vi "Practica_01.vi"() -> ()   [LabVIEW 2020]
panel:
  in  "stop":bool
  out "Grafica Filtro EMA":dbl(graph)
  out "Voltaje vs Tiempo":dbl[](graph)
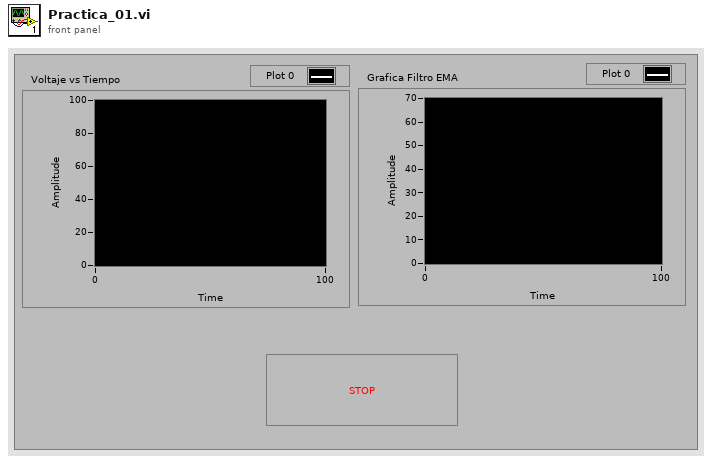
[diagram p1: front panel]
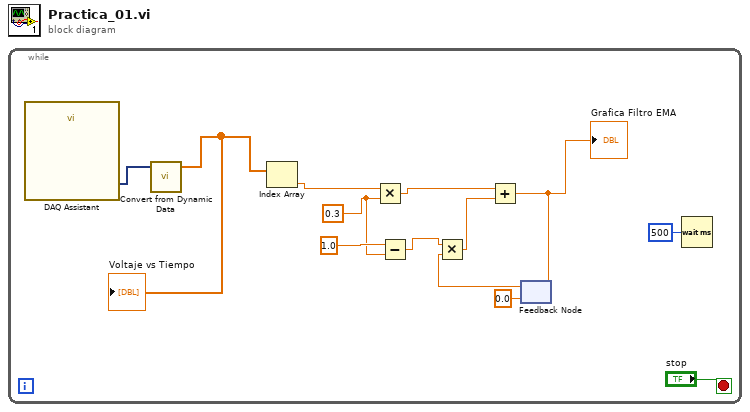
[diagram p0: block diagram]
diagram:
  n1 = while {
    stop <- "stop" stop-if-true
    w7 = 0.3 ("y")
    n2 = call "DAQ Assistant"() -> ("data"=w2:dynamicdata)  [unwired: 17 in, 2 out]
    n3 = call "Convert from Dynamic Data"("Dynamic Data Type"=w2) -> ("Array"=w1:dbl[])  [unwired: 3 in]
    "Voltaje vs Tiempo" <- w1
    n4 = Index Array(array=w1) -> (element=w3:dbl)  [unwired: 1 in]
    n5 = Multiply(x=w3, y=w7) -> (x*y=w11:dbl)
    n6 = Subtract(x=1.0, y=w7) -> (x-y=w9:dbl)
    n7 = feedback #1(0.0) -> (w6:dbl)
    n8 = Multiply(x=w9, y=w6) -> (x*y=w10:dbl)
    n9 = Add(x=w11, y=w10) -> (x+y=w4:dbl)
    "Grafica Filtro EMA" <- w4
    n10 = feedback-in #1(w4) -> ()
    n11 = Wait (ms)(milliseconds to wait=u32 500) -> ()  [unwired: 1 out]
  }
